vi "T90 Zustandsautomat.vi"(0 "Zustand":T2=enum."Warten", 1 "Modus:":T3=1 items=["Cal Gas", "Entnahmestelle"], 2 "Stabilisierungszeit":T1 format="%#_5g", 3 "Abweichung":T1 format="%#_5g", 4 "Sollwert":T1 format="%#_5g", 5 "IST-Wert":T1 format="%#_5g", 6 "Zeitstempel":timestamp, 8 "Abschaltzeit":T1 format="%#_5g") -> (16 "Timeout?":bool, 17 "Status":string, 18 "T50":dbl, 20 "Zustand":T2=enum."Warten", 21 "T90":dbl, 22 "T10":dbl, 23 "IST-Wert":T1 format="%#_5g", 24 "Rise time":dbl, 25 "Endwert":T1 format="%#_5g", 26 "Zeitstempel":timestamp, 27 "Signalverlauf":waveform(sgl) caption="Waveform")   [LabVIEW 2020, in "T90.lvlib"]
uses:
  T90.lvlib
  Aktion Zustandsautomat.ctl
  Zustand Auswahl.ctl
  Visualisierungs Elemente/Zahlen-Eingabefeld.ctl
  Aktion FGV T90.ctl
  Sprachverwaltung/FGV Aktion Tabelle zerlegen.ctl
  Seiten/CalGas Aufschaltung/FGV CalGas Aktionen.ctl
  Funktionstasten/Zustaende.ctl
  Funktionstasten/Funktionstasten-Aktion.ctl
  Seiten/CalGas Aufschaltung/Auswahl Aufschaltpunkt.ctl
  PNS/Aktionen FGV Grenzwerte.ctl
  Funktionstasten/Funktionstasten.lvlib
  Seiten/FT-IR/FT-IR.lvlib
  Allgemein/allgemeine Sub-VIs.lvlib
  Sprachverwaltung/Sprachverwaltung.lvlib
  Amium PNS/AK Kommunikation/AK Kommunikation.lvlib
  Amium PNS/AK Kommunikation/Amium Kommandos verwalten Aktionen.ctl
  PNS/PNS.lvlib
  Seiten/CalGas Aufschaltung/CalGas Aufschaltung.lvlib
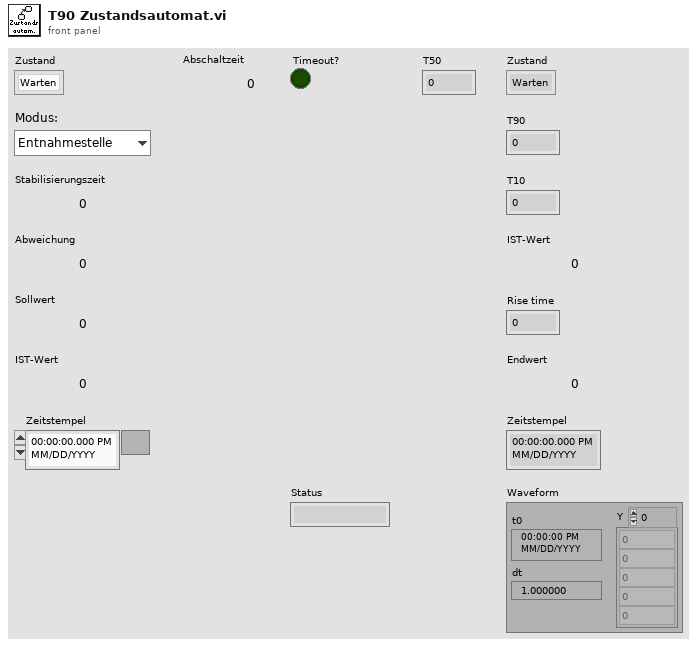
[diagram p1: front panel]
types:
  T1 = typedef "Zahlen-Eingabefeld.ctl" = sgl
  T2 = typedef "T90.lvlib/Aktion Zustandsautomat.ctl" = enum16{"Initialisieren", "Warten", "Gas aufschalten", "Stabilisieren", "Volle Konzentration 1", "Berechnen", "Prüfung starten", "Prüfung", "Prüfung beenden", "keine Funktion"}
  T3 = typedef "T90.lvlib/Zustand Auswahl.ctl" = u16
  T4 = typedef "CalGas Aufschaltung.lvlib/FGV CalGas Aktionen.ctl" = enum16{"lesen", "Analysator Auswahl", "Def.CalGas", "Aufschaltung CalGas", "laden", "speichern", "KAL extrahieren"}
  T5 = typedef "Sprachverwaltung.lvlib/FGV Aktion Tabelle zerlegen.ctl" = enum16{"laden", "vereinzeln", "speichern"}
  T6 = typedef "T90.lvlib/Aktion FGV T90.ctl" = enum16{"lesen", "schreiben", "laden", "speichern", "T90 aktiv", "T90 Entnahme aktiv", "Overflow Leak", "Pfad", "Zustand", "max. Responsetime"}
  T7 = typedef "Funktionstasten.lvlib/Funktionstasten-Aktion.ctl" = enum16{"Initialisieren", "Zustand setzen", "Taste gedrückt", "Fehler speichern", "Lesen", "Manuell", "Remote", "Bitparallel", "Samplepoint", "Zeit Prüfen", "reset Umschalten"}
  T8 = typedef "Funktionstasten.lvlib/Zustaende.ctl" = enum16{"Standby", "Pause", "Eco", "Messen", "Kalibrieren", "Spülen Filter", "Spülen Leitung", "Umgebungsluft", "0-Gas", "Cal-Gas", "CG zu PNS", "-------------", "Init 1", "Init 2", "Init 3", "Init 4", "Messen vorbereiten", "Messen durchführen", "Exit"}
  T9 = typedef "CalGas Aufschaltung.lvlib/Auswahl Aufschaltpunkt.ctl" = enum16{"über Filterblock", "Analysator direkt", "über PNS", "Entnahme", "Gasdivider"}
  T10 = typedef "PNS.lvlib/Aktionen FGV Grenzwerte.ctl" = enum16{"lesen", "Grenzw. schreiben", "Anweisungscode", "IP-Adresse", "laden", "speichern", "Anweisungscode vorgeben"}
  T11 = typedef "Amium PNS.lvlib/AK Kommunikation.lvlib/Amium Kommandos verwalten Aktionen.ctl" = enum16{"lesen", "setzen Ende", "setzen Pos1", "senden", "initalisieren", "prüfen", "Kommandos"}
  T12 = typedef "CalGas Aufschaltung.lvlib/Aufschaltung CalGas.ctl" = cluster{"Kalibriergas":T13, "Aufschaltpunkt":T9, "Analysator":T14}
  T13 = typedef "Auswahlfeld.ctl" = u16
  T14 = typedef "CalGas Aufschaltung.lvlib/Auswahl Analysator.ctl" = enum16{"FT-IR", "FID", "PMA", "PMA/FID/FT-IR"}
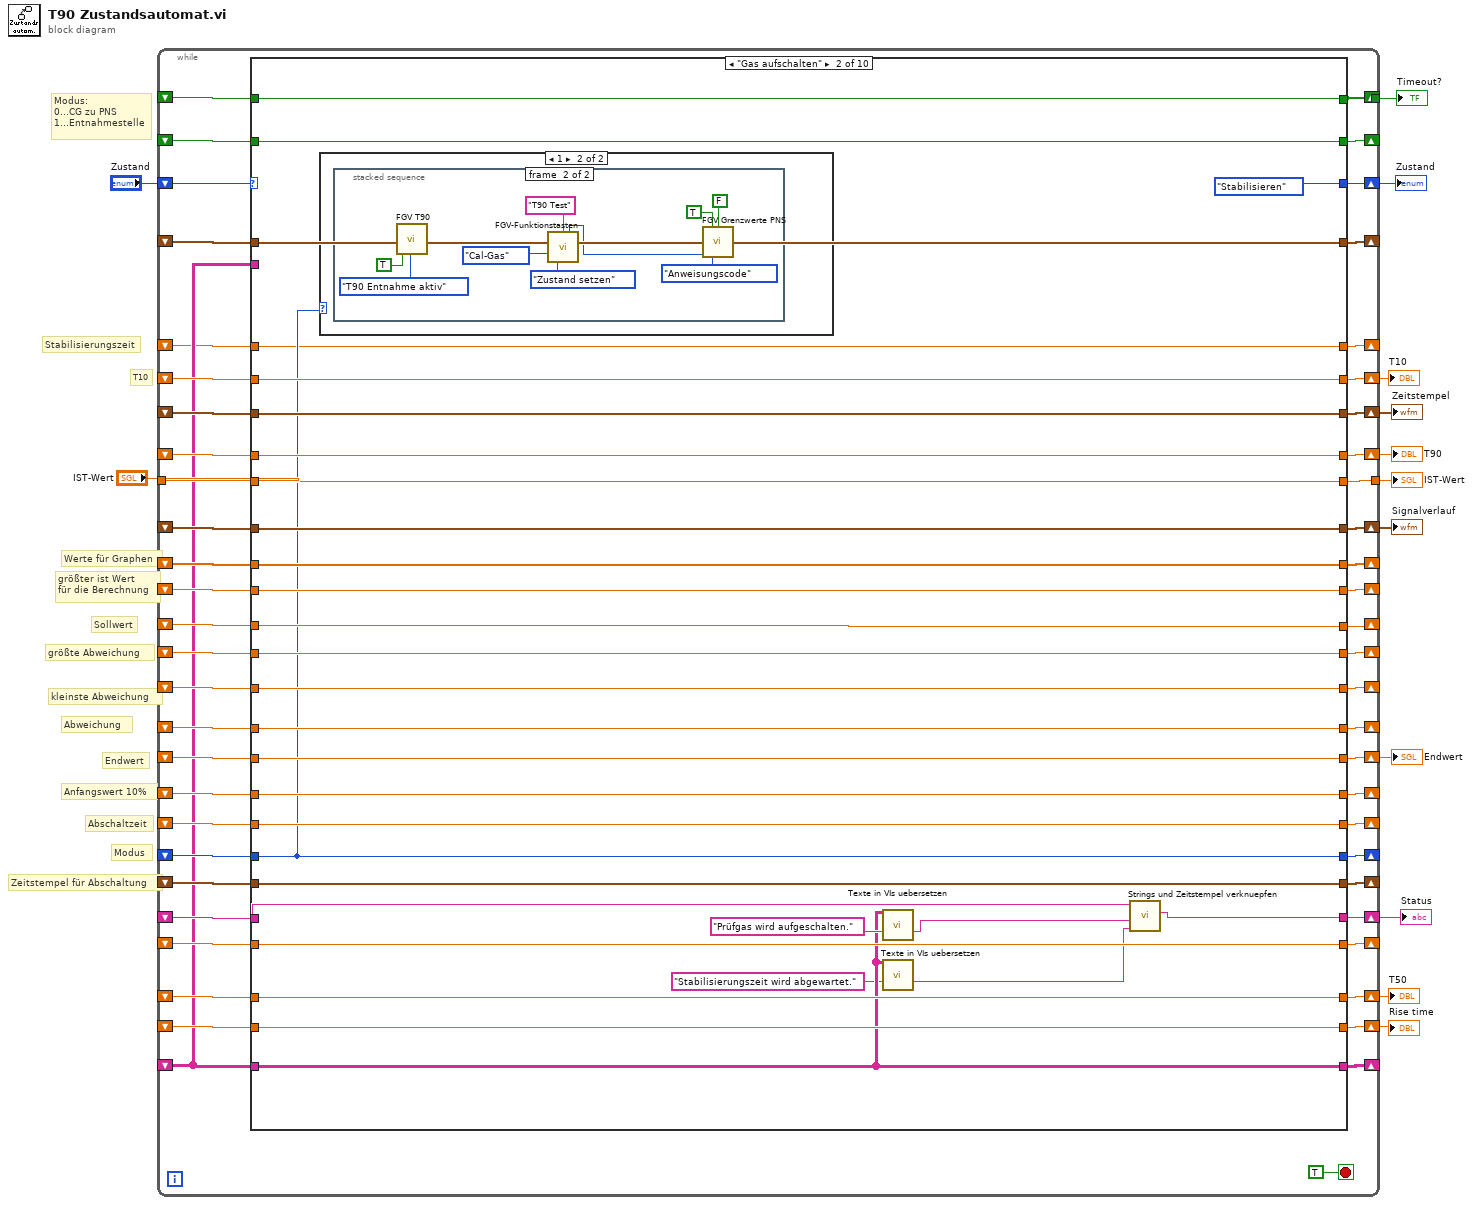
[diagram p0: block diagram]
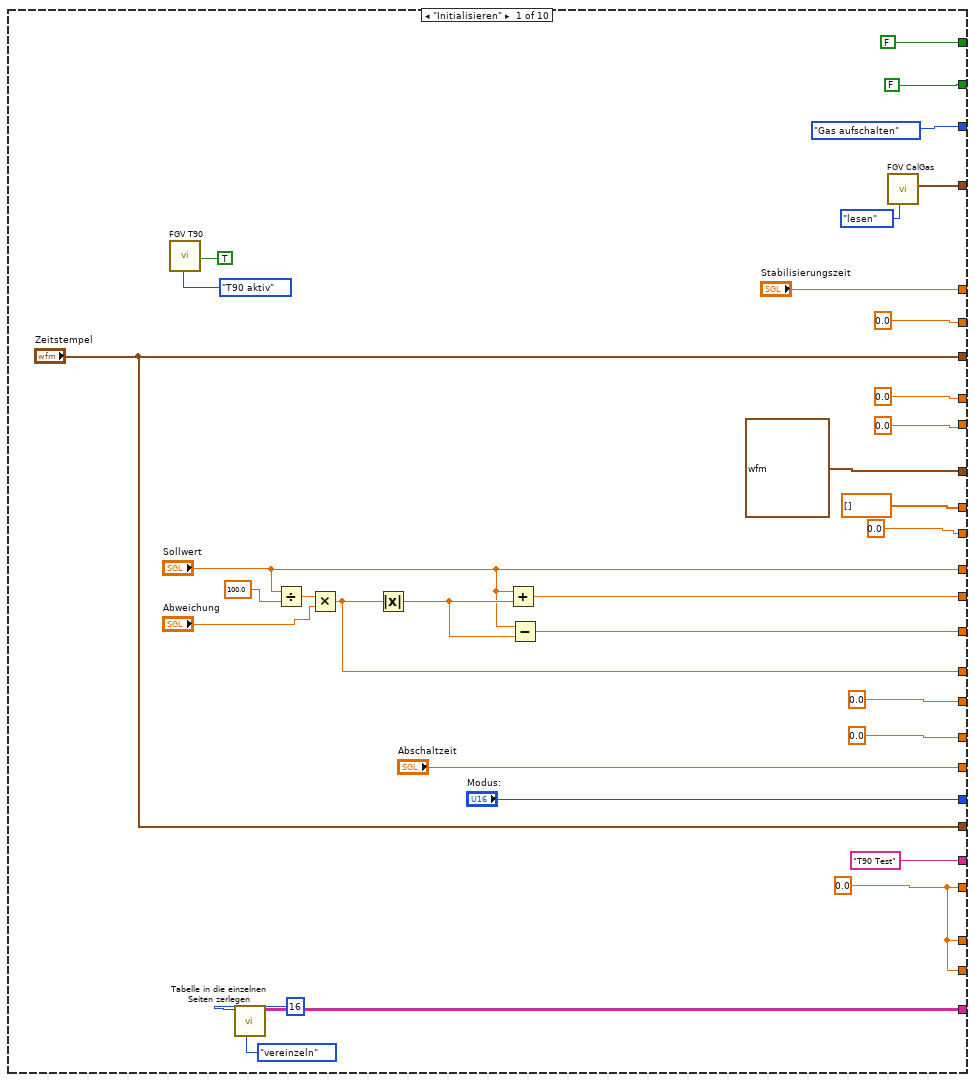
[diagram p2: hidden frame]
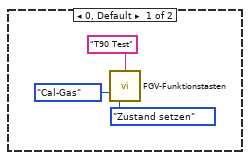
[diagram p3: hidden frame]
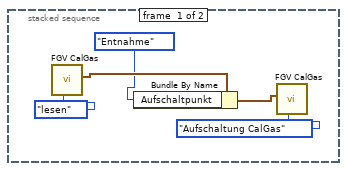
[diagram p4: hidden frame]
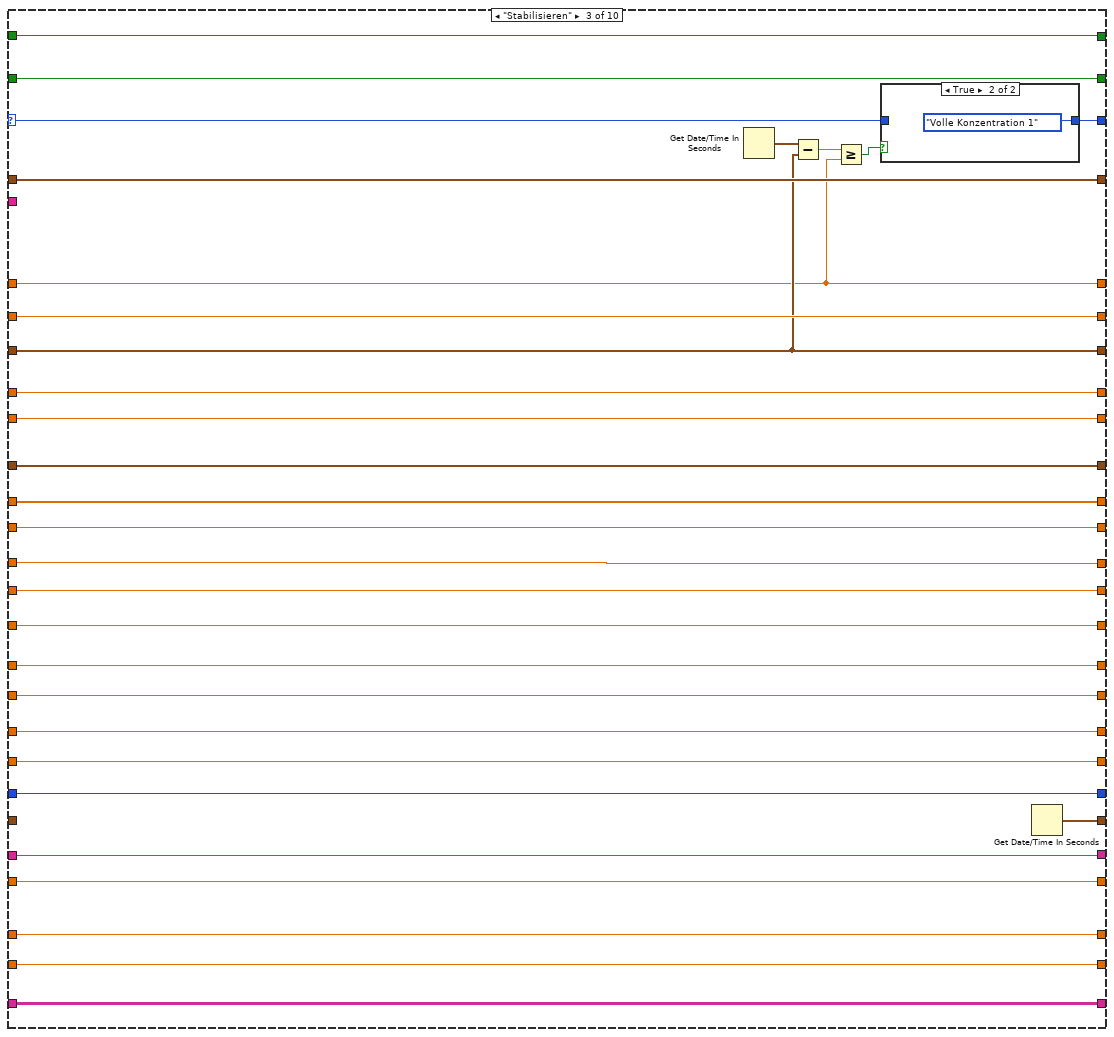
[diagram p5: hidden frame]
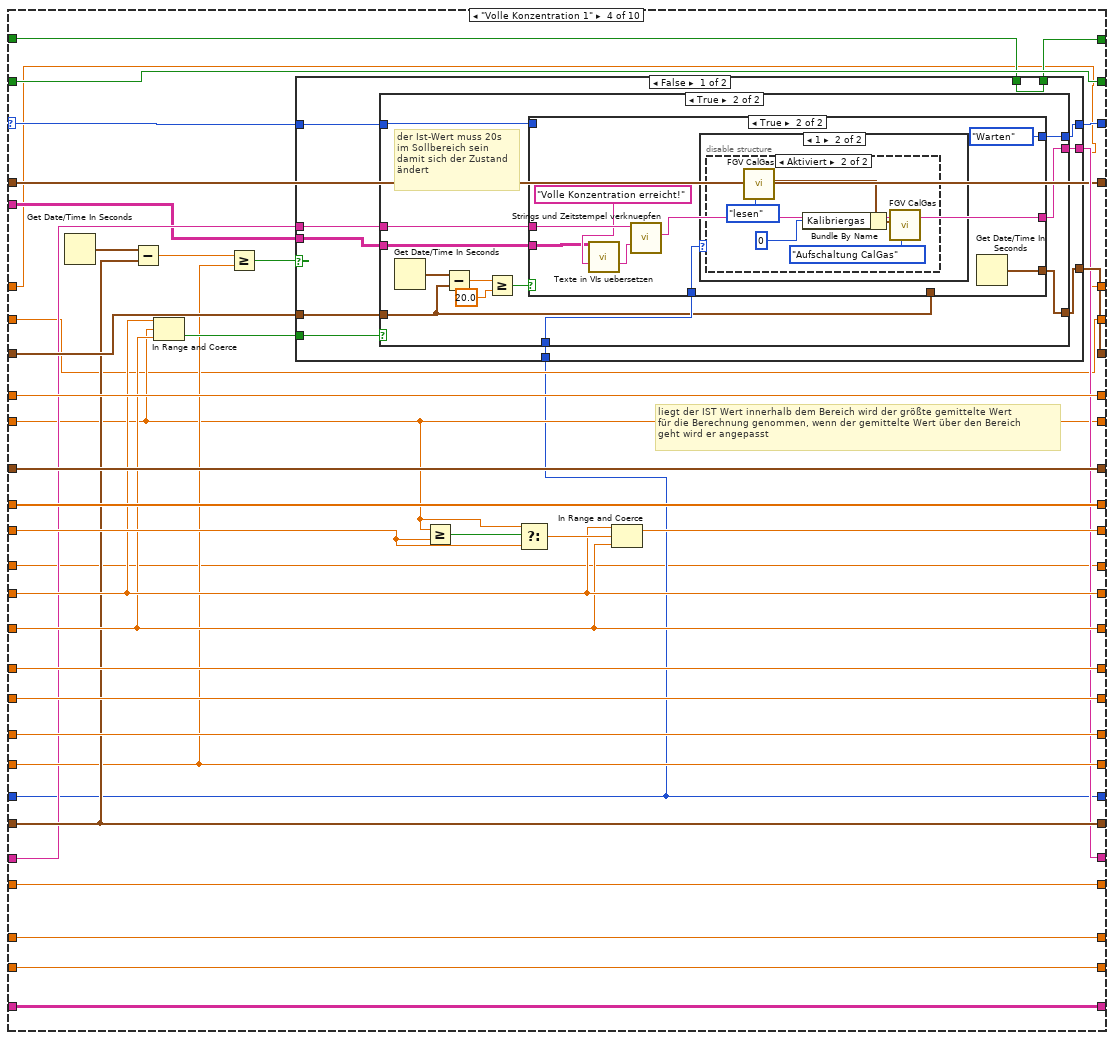
[diagram p7: hidden frame]
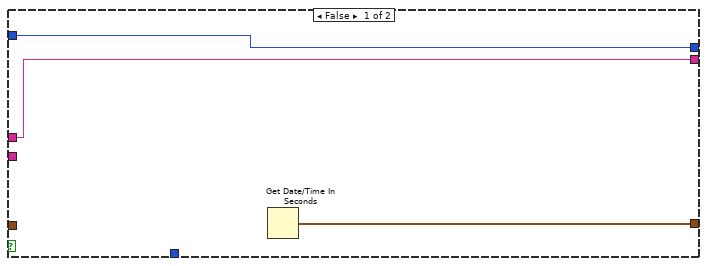
[diagram p8: hidden frame]
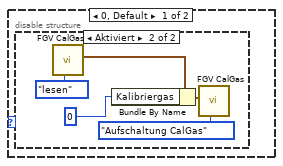
[diagram p10: hidden frame]
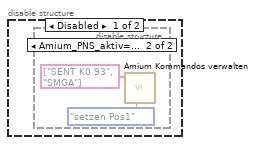
[diagram p11: hidden frame]
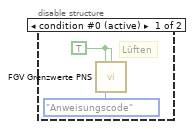
[diagram p12: hidden frame]
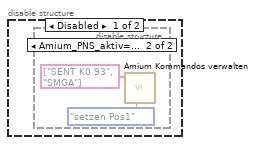
[diagram p13: hidden frame]
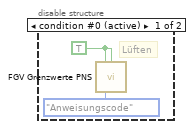
[diagram p14: hidden frame]
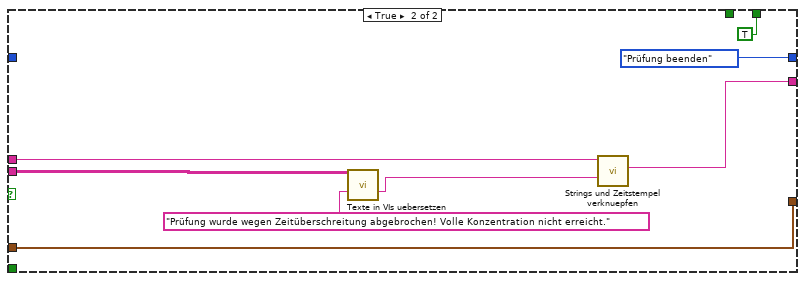
[diagram p15: hidden frame]
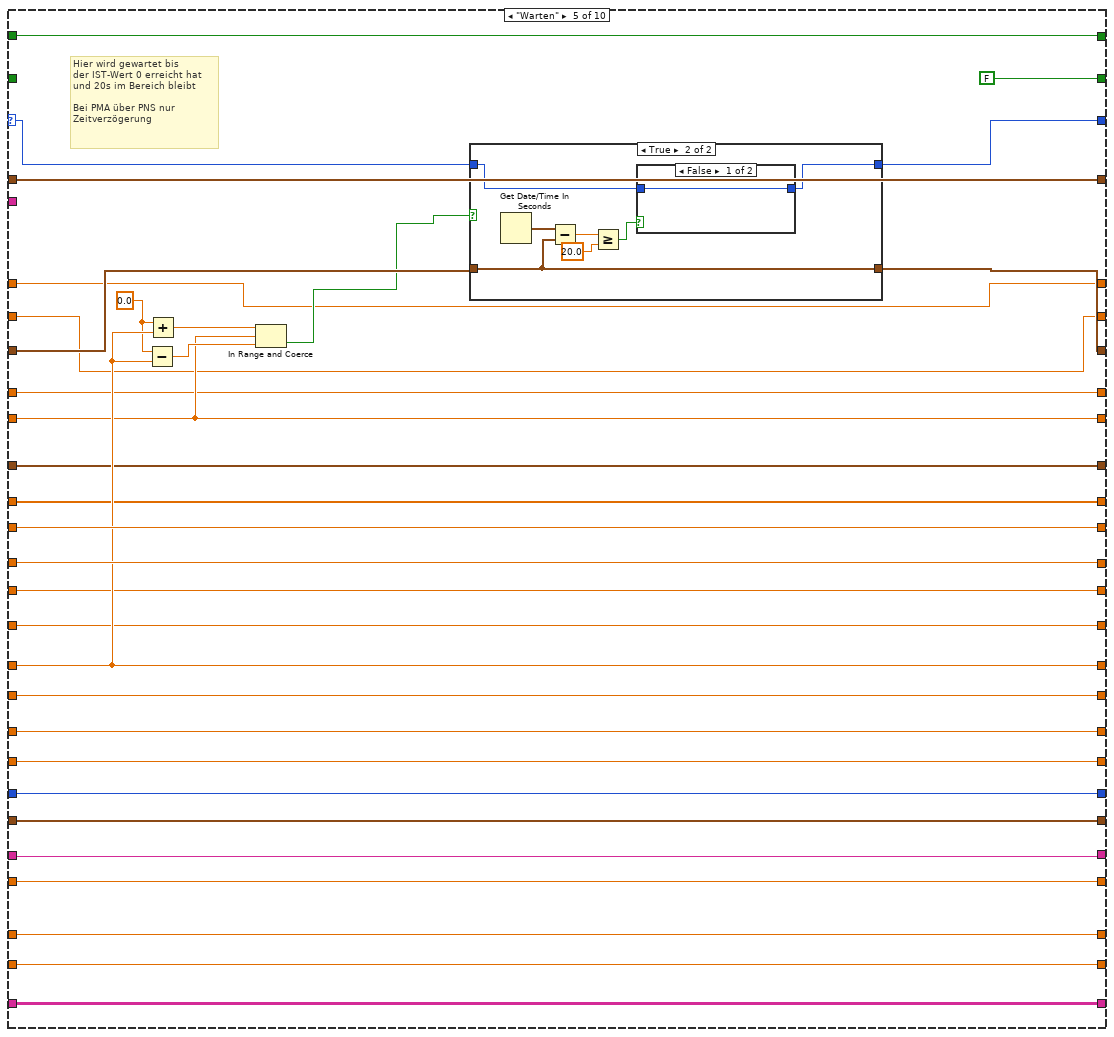
[diagram p16: hidden frame]
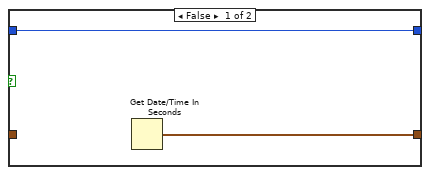
[diagram p17: hidden frame]
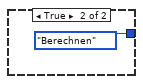
[diagram p18: hidden frame]
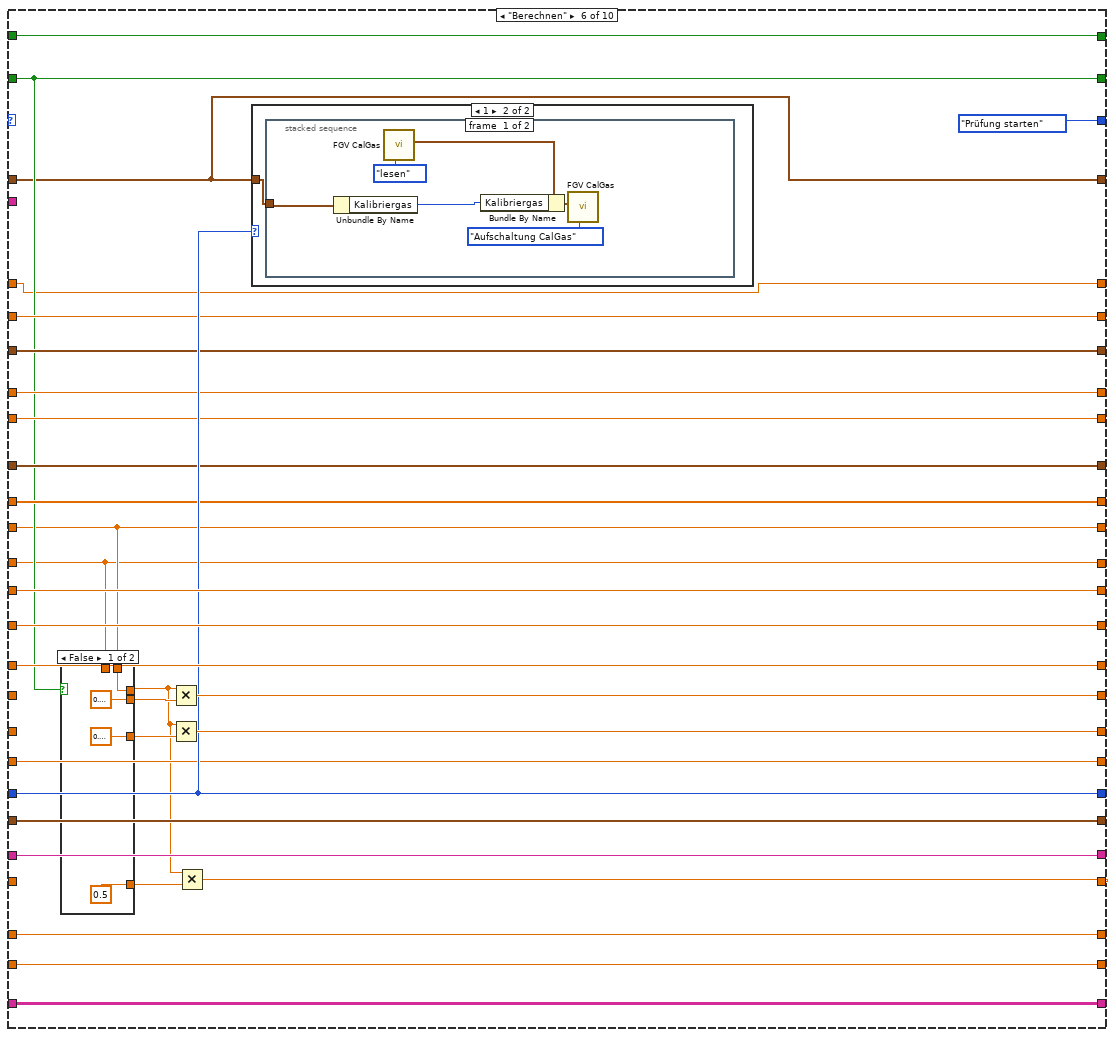
[diagram p19: hidden frame]
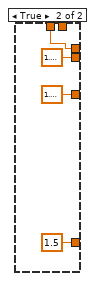
[diagram p20: hidden frame]
diagram:
  # "Stabilisierungszeit"
  # "Modus:\n0...CG zu PNS\n1...Entnahmestelle"
  # "T10"
  # "Zeitstempel für Abschaltung"
  # "Abschaltzeit"
  # "Werte für Graphen"
  # "Modus"
  # "größter ist Wert\nfür die Berechnung"
  # "Anfangswert 10%"
  # "Endwert"
  # "Abweichung"
  # "kleinste Abweichung"
  # "größte Abweichung"
  # "Sollwert"
  n1 = while {
    shift-right: [w61] -> _
    shift-left: _ -> [w63]
    shift-right: [w60] -> w8
    shift-left: _ -> [w59]
    tunnel: "IST-Wert" -> [w62]
    shift-right: [w58] -> _
    shift-left: _ -> [w56]
    shift-right: [w57] -> _
    shift-left: _ -> [w55]
    shift-right: [w64] -> w13
    shift-left: "Zustand" -> [w54]
    shift-right: [w53] -> _
    shift-left: _ -> [w52]
    shift-right: [w51] -> _
    shift-left: _ -> [w50]
    shift-right: [w49] -> w9
    shift-left: _ -> [w48]
    shift-right: [w47] -> _
    shift-left: _ -> [w46]
    shift-right: [w45] -> _
    shift-left: _ -> [w65]
    tunnel: [w43] -> w7
    shift-right: [w42] -> _
    shift-left: _ -> [w41]
    shift-right: [w40] -> w6
    shift-left: _ -> [w39]
    shift-right: [w44] -> w10
    shift-left: _ -> [w38]
    shift-right: [w37] -> _
    shift-left: _ -> [w36]
    shift-right: [w35] -> _
    shift-left: _ -> [w34]
    shift-right: [w33] -> w5
    shift-left: _ -> [w32]
    shift-right: [w31] -> w4
    shift-left: _ -> [w30]
    shift-right: [w29] -> _
    shift-left: _ -> [w28]
    shift-right: [w27] -> w3
    shift-left: _ -> [w26]
    shift-right: [w25] -> w2
    shift-left: _ -> [w24]
    shift-right: [w23] -> _
    shift-left: _ -> [w22]
    shift-right: [w21] -> _
    shift-left: _ -> [w20]
    shift-right: [w19] -> _
    shift-left: _ -> [w18]
    tunnel: [w16] -> w1
    shift-right: [w16] -> _
    shift-left: _ -> [w17]
    shift-right: [w15] -> _
    shift-left: _ -> [w14]
    stop <- TRUE stop-if-true
    n2 = case shown="\"Gas aufschalten\"" w54 {
      selector: w54 -> [_ _ w147 w212 w307 _ _ w451 _ w564]
      tunnel: w65 -> [_ w106 w155 w185 w301 w343 w398 w444 w536 w563]
      tunnel: [Aktion_Zustandsautomat."Gas aufschalten" ("Zustand") Aktion_Zustandsautomat."Stabilisieren" ("Zustand") w176 w213 w308 Aktion_Zustandsautomat."Prüfung starten" ("Zustand") Aktion_Zustandsautomat."Prüfung" ("Zustand") w450 Aktion_Zustandsautomat."keine Funktion" ("Zustand") w564] -> w64
      tunnel: w63 -> [_ w128 w175 w182 w304 w325 w404 w448 w533 w557]
      tunnel: w62 -> [_ w120 w168 w192 w296 w342 w396 w425 w527 _]
      tunnel: ["Sollwert" w128 w175 w182 w304 w325 w404 w448 w533 w557] -> w61
      tunnel: ["Zeitstempel" w127 w150 w215 w309 w337 w391 w429 w535 w562] -> w60
      tunnel: w59 -> [_ w127 w150 w214 w310 w337 _ w429 w535 w562]
      tunnel: [w97 w126 w174 w202 w298 w347 w403 w447 w532 w556] -> w58
      tunnel: [w96 w125 w173 w201 w297 w346 w402 w446 w531 w555] -> w57
      tunnel: w56 -> [_ w126 w174 w202 w298 w347 w403 w447 w532 w556]
      tunnel: w55 -> [_ w125 w173 w201 w297 w346 w402 w446 w531 w555]
      tunnel: [w78 w123 w171 w211 w299 w345 w401 w445 w530 w554] -> w53
      tunnel: w52 -> [_ w123 w171 w211 w299 w345 w401 w445 w530 w554]
      tunnel: [T1 0.0 ("IST-Wert") w124 w172 w200 w300 w326 w405 w449 w534 w558] -> w51
      tunnel: w50 -> [_ w124 w172 w209 w300 w326 w405 w449 w534 w558]
      tunnel: [T1 0.0 ("y") w122 w170 w208 w303 w350 w400 w424 w529 w553] -> w49
      tunnel: w48 -> [_ w122 w170 w208 w303 _ w400 w424 w529 w553]
      tunnel: [T1 0.0 ("y") w121 w169 w207 w302 w348 w399 w431 w528 w552] -> w47
      tunnel: w46 -> [_ w121 w169 w207 w302 _ w399 w431 w528 w552]
      tunnel: ["Modus:" w106 w155 w185 w301 w343 w398 w444 w536 w563] -> w45
      tunnel: [0.0 w117 w165 w204 w293 w339 w393 w412 w518 w551] -> w44
      tunnel: [T1 0.0 ("IST-Wert") w120 w168 w192 w296 w342 w396 w425 w527 T1 0.0 ("IST-Wert")] -> w43
      tunnel: [T1[] [] w118 w166 w205 w294 w341 w394 w443 w526 w559] -> w42
      tunnel: w41 -> [_ w118 w166 w205 w294 w341 w394 w442 w526 w559]
      tunnel: [waveform(sgl) {"t0"=timestamp(0 s since 1904-01-01), "dt"=1.0, "Y"=[]} w119 w167 w206 w295 w340 w395 w441 w525 w560] -> w40
      tunnel: w39 -> [_ w119 w167 w206 w295 w340 w395 _ w525 w560]
      tunnel: w38 -> [_ w117 w165 w204 w293 w339 w393 w426 w518 w551]
      tunnel: ["Abschaltzeit" w116 w164 w195 w292 w338 w392 w436 w523 w550] -> w37
      tunnel: w36 -> [_ w116 w164 w195 w292 w338 w392 w436 w523 w550]
      tunnel: ["Zeitstempel" w102 w163 w196 w291 w336 w391 w437 w522 w549] -> w35
      tunnel: w34 -> [_ w102 _ w196 w291 w336 _ w437 w522 w549]
      tunnel: ["T90 Test" w114 w162 w193 w280 w335 w389 w433 w521 w548] -> w33
      tunnel: w32 -> [_ w115 w162 w194 w280 w335 w390 w434 w521 w548]
      tunnel: [0.0 w113 w161 w191 w290 w334 w388 w411 w517 w547] -> w31
      tunnel: w30 -> [_ w113 w161 w191 w290 w334 w388 w432 w517 w547]
      tunnel: [w82 w112 w160 w190 w289 w332 w387 w428 w520 w546] -> w29
      tunnel: w28 -> [_ w112 w160 w190 w289 _ w387 w428 w520 w546]
      tunnel: [w82 w111 w159 w189 w288 w331 w386 w430 w519 w545] -> w27
      tunnel: w26 -> [_ w111 w159 w189 w288 w331 w386 w427 w519 w545]
      tunnel: [w82 w110 w158 w188 w287 w330 w385 w410 w511 w544] -> w25
      tunnel: w24 -> [_ w110 w158 w188 w287 w330 w385 _ w511 w544]
      tunnel: [w76 w101 w157 w187 w281 w329 w382 w423 w516 w543] -> w23
      tunnel: w22 -> [_ w101 w157 w187 w281 w329 w382 w423 w516 w543]
      tunnel: w22 -> [_ _ _ w186 _ _ _ w422 _ _]
      tunnel: [FALSE w107 w156 w184 FALSE w328 w381 w413 w513 w542] -> w21
      tunnel: w20 -> [_ w107 w156 w184 _ w328 w381 w413 w513 w542]
      tunnel: [w71 w105 w154 w183 w283 w324 w380 w409 w507 w541] -> w19
      tunnel: w18 -> [_ w105 w154 w183 w283 w324 w380 w409 w507 w541]
      tunnel: [FALSE w104 w153 w181 w282 w323 w379 w408 w506 w540] -> w16
      tunnel: w17 -> [_ w104 w153 w180 w282 w323 w379 w407 w506 w540]
      tunnel: ["Stabilisierungszeit" w103 w149 w179 w279 w322 w378 w406 w505 w539] -> w15
      tunnel: w14 -> [_ w103 w149 w179 w279 w322 w378 w406 w505 w539]
      frame "Initialisieren" {
        w82 = T1 0.0 ("y")
        n3 = call "FGV T90.vi"("aktiv"=TRUE, "Aktion"=Aktion_FGV_T90."T90 aktiv") -> ()  [unwired: 19 in, 7 out]
        n4 = call "Tabelle in die einzelnen Seiten zerlegen.vi"("Aktion"=FGV_Aktion_Tabelle_zerlegen."vereinzeln", "Index (Seite)"=16) -> ("Sprachliste"=w76:string[][])  [unwired: 7 in, 2 out]
        n5 = Divide(x="Sollwert", y=T1 100.0) -> (x/y=w80:T1)
        n6 = Multiply(x=w80, y="Abweichung") -> (x*y=w78:T1)
        n7 = Absolute Value(x=w78) -> (abs(x)=w98:T1)
        n8 = Add(x="Sollwert", y=w98) -> (x+y=w97:T1)
        n9 = Subtract(x="Sollwert", y=w98) -> (x-y=w96:T1)
        n10 = call "FGV CalGas.vi"("Aktionen"=FGV_CalGas_Aktionen."lesen") -> ("Aufschaltung CalGas"=w71:T12)  [unwired: 6 in, 4 out]
      }
      frame "Gas aufschalten" {
        n11 = case shown="1" w106 {
          frame 0, Default {
            n12 = call "FGV-Funktionstasten.vi"("Herkunft"="T90 Test", "Zustand"=Zustaende."Cal-Gas", "Aktion"=Funktionstasten-Aktion."Zustand setzen") -> ()  [unwired: 5 in, 8 out]
          }
          frame 1 {
            n13 = stacked-sequence {
              frame #0 {
                n14 = call "FGV CalGas.vi"("Aktionen"=FGV_CalGas_Aktionen."lesen") -> ("Aufschaltung CalGas"=w136:T12)  [unwired: 6 in, 4 out]
                n15 = Bundle By Name(cluster=w136, "Aufschaltpunkt"=Auswahl_Aufschaltpunkt."Entnahme") -> (w137:T12)
                n16 = call "FGV CalGas.vi"("Aktionen"=FGV_CalGas_Aktionen."Aufschaltung CalGas", "Aufschaltung CalGas"=w137) -> ()  [unwired: 5 in, 5 out]
              }
              frame #1 {
                n17 = call "FGV T90.vi"("Entnahme aktiv"=TRUE ("aktiv"), "Aktion"=Aktion_FGV_T90."T90 Entnahme aktiv") -> ()  [unwired: 19 in, 7 out]
                n18 = call "FGV-Funktionstasten.vi"("Herkunft"="T90 Test", "Zustand"=Zustaende."Cal-Gas", "Aktion"=Funktionstasten-Aktion."Zustand setzen") -> ("Samplepoint"=w138:u16)  [unwired: 5 in, 7 out]
                n19 = call "FGV Grenzwerte PNS.vi"("T90"=TRUE ("T90 lüften"), "T90 lüften"=FALSE, "Samplepoint"=w138, "Aktionen FGV Grenzwerte"=Aktionen_FGV_Grenzwerte."Anweisungscode") -> ()  [unwired: 9 in, 3 out]
              }
            }
          }
        }
        n20 = call "Texte in VIs uebersetzen.vi"("Sprachliste"=w101, "String zum Übersetzen"="Prüfgas wird aufgeschalten." ("String 1 hinzufügen")) -> ("String zum Übersetzen"=w108:string)  [unwired: 9 in, 4 out]
        n21 = call "Texte in VIs uebersetzen.vi"("Sprachliste"=w101, "String zum Übersetzen"="Stabilisierungszeit wird abgewartet." ("String 1 hinzufügen")) -> ("String zum Übersetzen"=w99:string)  [unwired: 9 in, 4 out]
        n22 = call "Strings und Zeitstempel verknuepfen.vi"("String 2 hinzufügen"=w99, "String 1 hinzufügen"=w108, "Eingagns String"=w115) -> ("Verknüpfter String"=w114:string)  [unwired: 8 in]
      }
      frame "Stabilisieren" {
        n23 = Get Date/Time In Seconds() -> (seconds since 1Jan1904=w152:timestamp)
        n24 = Subtract(x=w152, y=w150) -> (x-y=w151:dbl)
        n25 = Greater Or Equal?(x=w151, y=w149) -> (x >= y?=w148:bool)
        n26 = case shown="True" w148 {
          tunnel: [w177 Aktion_Zustandsautomat."Volle Konzentration 1" ("Zustand")] -> w176
          tunnel: w147 -> [w177 _]
          frame False {
          }
          frame True {
          }
        }
        n27 = Get Date/Time In Seconds() -> (seconds since 1Jan1904=w163:timestamp)
      }
      frame "Volle Konzentration 1" {
        # "liegt der IST Wert innerhalb dem Bereich wird der größte gemittelte Wert\nfür die Berechnung genommen, wenn der gemittelte Wert über den Bereich \ngeht wird er angepasst"
        n28 = Get Date/Time In Seconds() -> (seconds since 1Jan1904=w198:timestamp)
        n29 = Subtract(x=w198, y=w196) -> (x-y=w199:dbl)
        n30 = In Range and Coerce(upper limit=w202, x=w192, lower limit=w201) -> (In Range?=w216:bool)  [unwired: 1 out]
        n31 = Greater Or Equal?(x=w199, y=w195) -> (x >= y?=w197:bool)
        n32 = case shown="False" w197 {
          tunnel: w216 -> [w226 _]
          tunnel: [w225 w277] -> w215
          tunnel: w214 -> [w224 w277]
          tunnel: [w223 Aktion_Zustandsautomat."Prüfung beenden" ("Zustand")] -> w213
          tunnel: w212 -> [w222 _]
          tunnel: w194 -> [w221 w276]
          tunnel: [w220 w275] -> w193
          tunnel: w186 -> [w219 w272]
          tunnel: w185 -> [w218 _]
          tunnel: [w217 TRUE] -> w181
          tunnel: w180 -> [w217 _]
          frame False {
            n33 = case shown="True" w226 {
              tunnel: [w229 w230] -> w225
              tunnel: w224 -> [_ w231]
              tunnel: [w228 w237] -> w223
              tunnel: w222 -> [w228 w236]
              tunnel: w221 -> [w227 w235]
              tunnel: [w227 w234] -> w220
              tunnel: w219 -> [_ w233]
              tunnel: w218 -> [_ w232]
              frame False {
                n34 = Get Date/Time In Seconds() -> (seconds since 1Jan1904=w229:timestamp)
              }
              frame True {
                # "der Ist-Wert muss 20s\nim Sollbereich sein\ndamit sich der Zustand\nändert"
                n35 = Get Date/Time In Seconds() -> (seconds since 1Jan1904=w241:timestamp)
                n36 = Subtract(x=w241, y=w231) -> (x-y=w240:dbl)
                n37 = Greater Or Equal?(x=w240, y=20.0) -> (x >= y?=w238:bool)
                n38 = case shown="True" w238 {
                  tunnel: [w244 Aktion_Zustandsautomat."Warten" ("Zustand")] -> w237
                  tunnel: w236 -> [w244 _]
                  tunnel: w235 -> [w243 w251]
                  tunnel: [w243 w250] -> w234
                  tunnel: w233 -> [_ w248]
                  tunnel: w232 -> [_ w246]
                  tunnel: [w242 w245] -> w230
                  tunnel: w231 -> [w242 _]
                  frame False {
                  }
                  frame True {
                    n39 = call "Texte in VIs uebersetzen.vi"("Sprachliste"=w248, "String zum Übersetzen"="Volle Konzentration erreicht!" ("String 1 hinzufügen")) -> ("String zum Übersetzen"=w247:string)  [unwired: 9 in, 4 out]
                    n40 = call "Strings und Zeitstempel verknuepfen.vi"("String 1 hinzufügen"=w247, "Eingagns String"=w251) -> ("Verknüpfter String"=w250:string)  [unwired: 9 in]
                    n41 = case shown="1" w246 {
                      frame 0, Default {
                        n42 = disable-structure shown="Aktiviert" {
                          frame Disabled {
                            n43 = disable-structure shown="Amium_PNS_aktiv==TRUE" {
                              frame condition #0 (active) {
                                w253 = TRUE ("T90")
                                # "Lüften"
                                n44 = call "FGV Grenzwerte PNS.vi"("T90"=w253, "T90 lüften"=w253, "Aktionen FGV Grenzwerte"=Aktionen_FGV_Grenzwerte."Anweisungscode") -> ()  [unwired: 10 in, 3 out]
                              }
                              frame condition #1 {
                                n45 = call "Amium Kommandos verwalten.vi"("Aktionen"=Amium_Kommandos_verwalten_Aktionen."setzen Pos1", "neues Kommando Array"=string[] ["SENT K0 93", "SMGA"] ("neues Kommando")) -> ()  [unwired: 7 in, 3 out]
                              }
                            }
                          }
                          frame Enabled {
                            n46 = call "FGV CalGas.vi"("Aktionen"=FGV_CalGas_Aktionen."lesen") -> ("Aufschaltung CalGas"=w257:T12)  [unwired: 6 in, 4 out]
                            n47 = Bundle By Name(cluster=w257, "Kalibriergas"=0) -> (w259:T12)
                            n48 = call "FGV CalGas.vi"("Aktionen"=FGV_CalGas_Aktionen."Aufschaltung CalGas", "Aufschaltung CalGas"=w259) -> ()  [unwired: 5 in, 5 out]
                          }
                        }
                      }
                      frame 1 {
                        n49 = disable-structure shown="Aktiviert" {
                          frame Disabled {
                            n50 = disable-structure shown="Amium_PNS_aktiv==TRUE" {
                              frame condition #0 (active) {
                                w262 = TRUE ("T90")
                                # "Lüften"
                                n51 = call "FGV Grenzwerte PNS.vi"("T90"=w262, "T90 lüften"=w262, "Aktionen FGV Grenzwerte"=Aktionen_FGV_Grenzwerte."Anweisungscode") -> ()  [unwired: 10 in, 3 out]
                              }
                              frame condition #1 {
                                n52 = call "Amium Kommandos verwalten.vi"("Aktionen"=Amium_Kommandos_verwalten_Aktionen."setzen Pos1", "neues Kommando Array"=string[] ["SENT K0 93", "SMGA"] ("neues Kommando")) -> ()  [unwired: 7 in, 3 out]
                              }
                            }
                          }
                          frame Enabled {
                            n53 = call "FGV CalGas.vi"("Aktionen"=FGV_CalGas_Aktionen."lesen") -> ("Aufschaltung CalGas"=w266:T12)  [unwired: 6 in, 4 out]
                            n54 = Bundle By Name(cluster=w266, "Kalibriergas"=0) -> (w268:T12)
                            n55 = call "FGV CalGas.vi"("Aktionen"=FGV_CalGas_Aktionen."Aufschaltung CalGas", "Aufschaltung CalGas"=w268) -> ()  [unwired: 5 in, 5 out]
                          }
                        }
                      }
                    }
                    n56 = Get Date/Time In Seconds() -> (seconds since 1Jan1904=w245:timestamp)
                  }
                }
              }
            }
          }
          frame True {
            n57 = call "Texte in VIs uebersetzen.vi"("Sprachliste"=w272, "String zum Übersetzen"="Prüfung wurde wegen Zeitüberschreitung abgebrochen! Volle Konzentration nicht erreicht." ("String 1 hinzufügen")) -> ("String zum Übersetzen"=w273:string)  [unwired: 9 in, 4 out]
            n58 = call "Strings und Zeitstempel verknuepfen.vi"("String 1 hinzufügen"=w273, "Eingagns String"=w276) -> ("Verknüpfter String"=w275:string)  [unwired: 9 in]
          }
        }
        n59 = Greater Or Equal?(x=w192, y=w209) -> (x >= y?=w210:bool)
        n60 = Select(t=w192, s=w210, f=w209) -> (s? t:f=w203:T1)
        n61 = In Range and Coerce(upper limit=w202, x=w203, lower limit=w201) -> (coerced(x)=w200:T1)  [unwired: 1 out]
      }
      frame "Warten" {
        w286 = T1 0.0 ("x")
        # "Hier wird gewartet bis\nder IST-Wert 0 erreicht hat und 20s im Bereich bleibt\n\nBei PMA über PNS nur Zeitverzögerung"
        n62 = Subtract(x=w286, y=w299) -> (x-y=w305:T1)
        n63 = Add(x=w286, y=w299) -> (x+y=w306:T1)
        n64 = In Range and Coerce(upper limit=w306, x=w296, lower limit=w305) -> (In Range?=w285:bool)  [unwired: 1 out]
        n65 = case shown="True" w285 {
          tunnel: [w312 w319] -> w309
          tunnel: w310 -> [_ w319]
          tunnel: [w311 w314] -> w308
          tunnel: w307 -> [w311 w313]
          frame False {
            n66 = Get Date/Time In Seconds() -> (seconds since 1Jan1904=w312:timestamp)
          }
          frame True {
            n67 = Get Date/Time In Seconds() -> (seconds since 1Jan1904=w318:timestamp)
            n68 = Subtract(x=w318, y=w319) -> (x-y=w317:dbl)
            n69 = Greater Or Equal?(x=w317, y=20.0) -> (x >= y?=w315:bool)
            n70 = case shown="False" w315 {
              tunnel: [w320 Aktion_Zustandsautomat."Berechnen" ("Zustand")] -> w314
              tunnel: w313 -> [w320 _]
              frame False {
              }
              frame True {
              }
            }
          }
        }
      }
      frame "Berechnen" {
        n71 = case shown="False" w328 {
          tunnel: [T1 0.9 ("y") T1 1.1 ("y")] -> w351
          tunnel: [T1 0.1 ("y") T1 1.9 ("y")] -> w349
          tunnel: [T1 0.5 ("y") T1 1.5 ("y")] -> w333
          tunnel: [w352 w356] -> w327
          tunnel: w326 -> [w352 _]
          tunnel: w325 -> [_ w356]
          frame False {
          }
          frame True {
          }
        }
        n72 = Multiply(x=w327, y=w351) -> (x*y=w350:T1)
        n73 = Multiply(x=w327, y=w349) -> (x*y=w348:T1)
        n74 = Multiply(x=w327, y=w333) -> (x*y=w332:T1)
        n75 = case shown="1" w343 {
          tunnel: w324 -> [w360 w362]
          frame 0, Default {
            n76 = call "FGV CalGas.vi"("Aktionen"=FGV_CalGas_Aktionen."Aufschaltung CalGas", "Aufschaltung CalGas"=w360) -> ()  [unwired: 5 in, 5 out]
          }
          frame 1 {
            n77 = stacked-sequence {
              tunnel: w362 -> [w366 _]
              frame #0 {
                n78 = Unbundle By Name(w366) -> ("Kalibriergas"=w365:T13)
                n79 = call "FGV CalGas.vi"("Aktionen"=FGV_CalGas_Aktionen."lesen") -> ("Aufschaltung CalGas"=w363:T12)  [unwired: 6 in, 4 out]
                n80 = Bundle By Name(cluster=w363, "Kalibriergas"=w365) -> (w367:T12)
                n81 = call "FGV CalGas.vi"("Aktionen"=FGV_CalGas_Aktionen."Aufschaltung CalGas", "Aufschaltung CalGas"=w367) -> ()  [unwired: 5 in, 5 out]
              }
              frame #1 {
                n82 = call "FGV T90.vi"("Entnahme aktiv"=TRUE ("aktiv"), "Aktion"=Aktion_FGV_T90."T90 Entnahme aktiv") -> ()  [unwired: 19 in, 7 out]
                n83 = call "FGV-Funktionstasten.vi"("Herkunft"="T90 Test", "Zustand"=Zustaende."Cal-Gas", "Aktion"=Funktionstasten-Aktion."Zustand setzen") -> ("Samplepoint"=w369:u16)  [unwired: 5 in, 7 out]
                n84 = call "FGV Grenzwerte PNS.vi"("T90"=TRUE ("T90 lüften"), "T90 lüften"=FALSE, "Samplepoint"=w369, "Aktionen FGV Grenzwerte"=Aktionen_FGV_Grenzwerte."Anweisungscode") -> ()  [unwired: 9 in, 3 out]
              }
            }
          }
        }
      }
      frame "Prüfung starten" {
        n85 = call "Texte in VIs uebersetzen.vi"("Sprachliste"=w382, "String zum Übersetzen"="Prüfung wird gestartet." ("String 1 hinzufügen")) -> ("String zum Übersetzen"=w383:string)  [unwired: 9 in, 4 out]
        n86 = Get Date/Time In Seconds() -> (seconds since 1Jan1904=w391:timestamp)
        n87 = call "Strings und Zeitstempel verknuepfen.vi"("String 1 hinzufügen"=w383, "Eingagns String"=w390) -> ("Verknüpfter String"=w389:string)  [unwired: 9 in]
      }
      frame "Prüfung" {
        # "0,2 = Timing der Schleife \n          bei T90 main.vi"
        n88 = Get Date/Time In Seconds() -> (seconds since 1Jan1904=w438:timestamp)
        n89 = Subtract(x=w438, y=w437) -> (x-y=w439:dbl)
        n90 = Greater Or Equal?(x=w439, y=w436) -> (x >= y?=w435:bool)
        n91 = Greater Or Equal?(x=w425, y=w424) -> (x >= y?=w414:bool)
        n92 = case shown="True" w413 {
          tunnel: [w452 w453] -> w415
          tunnel: w414 -> [w452 w454]
          frame False {
          }
          frame True {
            n93 = Not(x=w454) -> (.not. x?=w453:bool)
          }
        }
        n94 = case shown="True" w435 {
          tunnel: w415 -> [w479 _]
          tunnel: w451 -> [w484 _]
          tunnel: [w483 Aktion_Zustandsautomat."Prüfung beenden" ("Zustand")] -> w450
          tunnel: w434 -> [w482 w503]
          tunnel: [w481 w502] -> w433
          tunnel: w422 -> [w477 w499]
          tunnel: [w476 TRUE] -> w408
          tunnel: w407 -> [w476 _]
          frame False {
            n95 = disable-structure shown="Deaktiviert" {
              disable-tunnel: [w488 w489] -> w480
              disable-tunnel: w479 -> [w487 w489]
              disable-tunnel: FALSE ("Abfallverzögerung?") -> [w486 _]
              frame Disabled {
                n96 = call "Verzoegerung PC.vi"("Abfallverzögerung?"=w486, "sec"=u16 5, "Startsignal"=w487) -> ("Zeit abgelaufen?"=w488:bool)  [unwired: 7 in, 1 out]
              }
              frame Enabled {
              }
            }
            n97 = case shown="False" w480 {
              tunnel: [w491 Aktion_Zustandsautomat."Prüfung beenden" ("Zustand")] -> w483
              tunnel: w484 -> [w491 _]
              tunnel: w482 -> [w490 w496]
              tunnel: [w490 w495] -> w481
              tunnel: w477 -> [_ w492]
              frame False {
              }
              frame True {
                n98 = call "Texte in VIs uebersetzen.vi"("Sprachliste"=w492, "String zum Übersetzen"="Prüfung wurde beendet!" ("String 1 hinzufügen")) -> ("String zum Übersetzen"=w493:string)  [unwired: 9 in, 4 out]
                n99 = call "Strings und Zeitstempel verknuepfen.vi"("String 1 hinzufügen"=w493, "Eingagns String"=w496) -> ("Verknüpfter String"=w495:string)  [unwired: 9 in]
              }
            }
          }
          frame True {
            n100 = call "Texte in VIs uebersetzen.vi"("Sprachliste"=w499, "String zum Übersetzen"="Prüfung wurde wegen einer Zeitüberschreitung abgebrochen!" ("String 1 hinzufügen")) -> ("String zum Übersetzen"=w500:string)  [unwired: 9 in, 4 out]
            n101 = call "Strings und Zeitstempel verknuepfen.vi"("String 1 hinzufügen"=w500, "Eingagns String"=w503) -> ("Verknüpfter String"=w502:string)  [unwired: 9 in]
          }
        }
        n102 = Greater Or Equal?(x=w425, y=w431) -> (x >= y?=w421:bool)
        n103 = Greater Or Equal?(x=w425, y=w424) -> (x >= y?=w419:bool)
        n104 = Greater Or Equal?(x=w425, y=w428) -> (x >= y?=w416:bool)
        n105 = case shown="True" w413 {
          tunnel: w421 -> [w459 w463]
          tunnel: [w459 w461] -> w420
          tunnel: w419 -> [w458 w462]
          tunnel: [w458 w460] -> w418
          frame False {
          }
          frame True {
            n106 = Not(x=w463) -> (.not. x?=w461:bool)
            n107 = Not(x=w462) -> (.not. x?=w460:bool)
          }
        }
        n108 = case shown="True" w413 {
          tunnel: [w455 w456] -> w417
          tunnel: w416 -> [w455 w457]
          frame False {
          }
          frame True {
            n109 = Not(x=w457) -> (.not. x?=w456:bool)
          }
        }
        n110 = case shown="False" w420 {
          tunnel: w429 -> [w473 _]
          tunnel: [w472 w475] -> w411
          tunnel: w432 -> [_ w475]
          frame False {
            # "T10"
            n111 = Get Date/Time In Seconds() -> (seconds since 1Jan1904=w474:timestamp)
            n112 = Subtract(x=w474, y=w473) -> (x-y=w472:dbl)
          }
          frame True {
          }
        }
        n113 = case shown="False" w418 {
          tunnel: [w465 w467] -> w412
          tunnel: w429 -> [w464 _]
          tunnel: w426 -> [_ w467]
          frame False {
            n114 = Get Date/Time In Seconds() -> (seconds since 1Jan1904=w466:timestamp)
            n115 = Subtract(x=w466, y=w464) -> (x-y=w465:dbl)
          }
          frame True {
          }
        }
        n116 = case shown="False" w417 {
          tunnel: [w469 w471] -> w430
          tunnel: w427 -> [_ w471]
          tunnel: w429 -> [w468 _]
          frame False {
            # "T50"
            n117 = Get Date/Time In Seconds() -> (seconds since 1Jan1904=w470:timestamp)
            n118 = Subtract(x=w470, y=w468) -> (x-y=w469:dbl)
          }
          frame True {
          }
        }
        n119 = Bundle By Name("dt"=0.2, "t0"=w429, "Y"=w442) -> (w441:waveform(sgl))  [unwired: 1 in]
        n120 = Subtract(x=w412, y=w411) -> (x-y=w410:dbl)
        n121 = Build Array (concatenate)(w442, w425) -> (w443:T1[])
      }
      frame "Prüfung beenden" {
        n122 = call "FGV T90.vi"("aktiv"=FALSE, "Aktion"=Aktion_FGV_T90."T90 aktiv") -> ()  [unwired: 19 in, 7 out]
        n123 = call "FGV CalGas.vi"("Aktionen"=FGV_CalGas_Aktionen."Aufschaltung CalGas", "Aufschaltung CalGas"=w507) -> ()  [unwired: 5 in, 5 out]
        n124 = call "FGV-Funktionstasten.vi"("Herkunft"="T90 Test", "Zustand"=Zustaende."Standby", "Aktion"=Funktionstasten-Aktion."Zustand setzen") -> ()  [unwired: 5 in, 8 out]
        n125 = call "FGV T90.vi"("Entnahme aktiv"=FALSE ("aktiv"), "Aktion"=Aktion_FGV_T90."T90 Entnahme aktiv") -> ()  [unwired: 19 in, 7 out]
      }
      frame "keine Funktion" {
      }
    }
  }
  "Zustand" <- w13
  "T90" <- w10
  "Endwert" <- w9
  "Zeitstempel" <- w8
  "IST-Wert" <- w7
  "Signalverlauf" <- w6
  "Status" <- w5
  "T10" <- w4
  "T50" <- w3
  "Rise time" <- w2
  "Timeout?" <- w1
